vi "TestCode.vi"   [LabVIEW 2020]
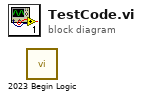
[diagram p0: block diagram]
diagram:
  n1 = call "2023 Begin Logic.vi"() -> ()  [unwired: 1 in, 1 out]
